vi "Unflatten Shared Resources.vi"(8 "error in":errorcluster, 11 "flattened shared resources":string) -> (0 "error out":errorcluster, 3 "shared resources":refnum<class "Shared Resources.lvclass">)   [LabVIEW 2020, in "Communication Bus Template Engine.lvlib" / "Custom Device.lvlib"]
uses:
  Custom Device.lvlib
  Interfaces/Shared Resources/Shared Resources.lvclass
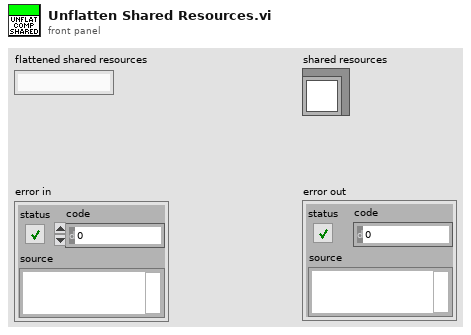
[diagram p1: front panel]
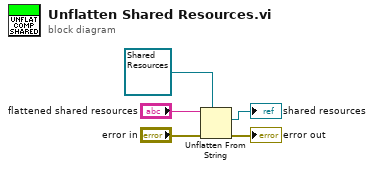
[diagram p0: block diagram]
diagram:
  n1 = Unflatten From String(type=refnum<class "Shared Resources.lvclass"> refnum ("Shared Resources"), binary string="flattened shared resources", error in (no error)="error in") -> (value=→"shared resources":refnum<class "Shared Resources.lvclass">, error out=→"error out":errorcluster)  [unwired: 2 in, 1 out]
